vi "ZSort_Scan_Params.vi"(8 "error in (no error)":errorcluster, 11 "Sweep Metadata Cluster":T1 {"Channels: AO"."AO f (Hz)" min=0.001 max=10000.0; "Channels: AO"."AO DC (V)" format="%#_6p"; "Channels: AO"."AO amp (V)" format="%#_6p"}) -> (0 "error out":errorcluster, 1 "Sorted scan parameters":cluster{T15}[](array[cluster])=[{[{"Start"=0.14, "End"=-0.060000000000000005, "Step"=-0.060000000000000005, "Rate"=0.0, "wait (ms)"=10000, "address"="\nscaledVsg1=", "Channel"=2}]}, {[{"Start"=0.14, "End"=-0.060000000000000005, "Step"=-0.060000000000000005, "Rate"=0.0, "wait (ms)"=10000, "address"="\nscaledVsg1=", "Channel"=2}]}, {[{"Start"=0.14, "End"=-0.060000000000000005, "Step"=-0.060000000000000005, "Rate"=0.0, "wait (ms)"=10000, "address"="\nscaledVsg1=", "Channel"=2}, {"Start"=0.14, "End"=-0.060000000000000005, "Step"=-0.060000000000000005, "Rate"=0.0, "wait (ms)"=10000, "address"="\nscaledVsg1=", "Channel"=3}]}] {"?"."Rate" format="%.2f"; "?"."Step" format="%#_6p"; "?"."End" format="%#_6p"; "?"."Start" format="%#_6p"}, 2 "Sorted scan control":cluster{T11}[](array[cluster])=[{[{"Priority"=enum."Priority 0", "Scan name"=enum."DSA_Vsg2"}]}, {[{"Priority"=enum."Priority 1", "Scan name"=enum."DSA_Vamp"}]}, {[{"Priority"=enum."Priority 2", "Scan name"=enum."DSA_Vsg1"}, {"Priority"=enum."Priority 2", "Scan name"=enum."DSA_Vsg3"}]}])   [LabVIEW 2016]
uses:
  levylab_expt_transport/src/SMOs/SweepControl/Typedefs/Cluster - ScanParamters.ctl
  levylab_expt_transport/src/SMOs/SweepControl/SweepControl.lvclass
  levylab_expt_transport/src/SMOs/SweepControl/Typedefs/ScanParamters.ctl
  levylab_expt_transport/src/SMOs/SweepControl/Typedefs/Enum - Priority.ctl
  levylab_expt_transport/src/SMOs/SweepControl/Typedefs/Enum - Action.ctl
  levylab_expt_transport/src/SMOs/SweepControl/Typedefs/Cluster - ScanControl.ctl
  levylab_expt_transport/src/SMOs/SweepControl/Typedefs/ScanControl.ctl
  <userlib>/LevyLab/Lockin-Multichannel/Typedefs/AO_Amp-array.ctl
  <userlib>/LevyLab/Lockin-Multichannel/Typedefs/AO_DC-array.ctl
  <userlib>/LevyLab/Lockin-Multichannel/Typedefs/AO_phi-array.ctl
  <userlib>/LevyLab/Lockin-Multichannel/Typedefs/Function-enum.ctl
  <userlib>/LevyLab/Lockin-Multichannel/Typedefs/Function-array.ctl
  <userlib>/LevyLab/Lockin-Multichannel/Typedefs/AO_f-array.ctl
  <userlib>/LevyLab/Lockin-Multichannel/Typedefs/AO-cluster.ctl
  levylab_expt_transport/src/SMOs/SweepControl/Typedefs/Enum - PostAction.ctl
  levylab_expt_transport/src/SMOs/SweepControl/Typedefs/PostAction.ctl
  levylab_expt_transport/src/subVI/SweepMetadataV2.ctl
panel:
  # "0"
  # "1"
  # "2"
  # "3"
  # "4"
  # "5"
  # "6"
  # "7"
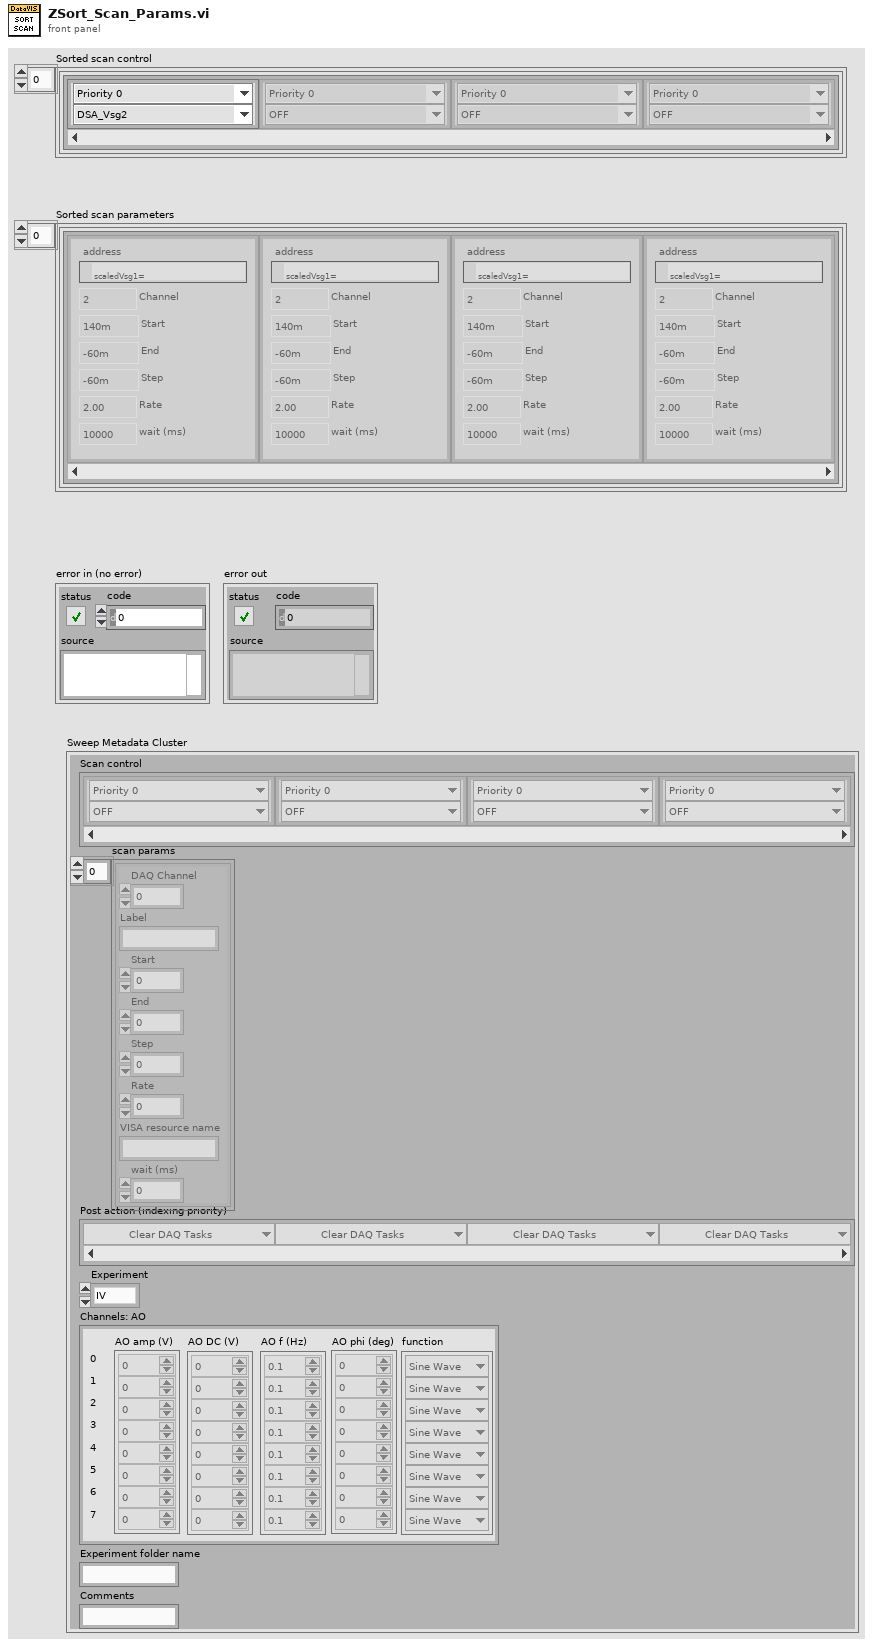
[diagram p1: front panel]
types:
  T1 = typedef "SweepMetadataV2.ctl" = cluster{"Experiment":enum16{"IV", "lockin_time", "Lockin_Vsg"}, "Experiment folder name":string, "Comments":string, "Channels: AO":T2, "Post action (indexing priority)":T9, "Scan control":T11, "scan params":cluster{"DAQ Channel":i32, "Label":string, "Start":dbl, "End":dbl, "Step":dbl, "Rate":dbl, "VISA resource name":string, "wait (ms)":u32}[]}
  T2 = typedef "AO-cluster.ctl" = cluster{"AO amp (V)":T3, "AO DC (V)":T4, "AO f (Hz)":T5, "AO phi (deg)":T6, "function":T7}
  T3 = typedef "AO_Amp-array.ctl" = dbl[]
  T4 = typedef "AO_DC-array.ctl" = dbl[]
  T5 = typedef "AO_f-array.ctl" = dbl[]
  T6 = typedef "AO_phi-array.ctl" = dbl[]
  T7 = typedef "Function-array.ctl" = T8[]
  T8 = typedef "Function-enum.ctl" = enum16{"Sine Wave", "Triangle Wave", "Square Wave", "Sawtooth Wave"}
  T9 = typedef "SweepControl.lvclass/PostAction.ctl" = T10[]
  T10 = typedef "SweepControl.lvclass/Enum - PostAction.ctl" = enum16{"Clear DAQ Tasks", "Check Temperature", "Wait", "Do Nothing"}
  T11 = typedef "SweepControl.lvclass/ScanControl.ctl" = T12[]
  T12 = typedef "SweepControl.lvclass/Cluster - ScanControl.ctl" = cluster{"Priority":T13, "Scan name":T14}
  T13 = typedef "SweepControl.lvclass/Enum - Priority.ctl" = enum16{"Priority 0", "Priority 1", "Priority 2", "Priority 3", "Priority 4", "Priority 5"}
  T14 = typedef "SweepControl.lvclass/Enum - Action.ctl" = enum16{"OFF", "DSA_Vamp", "DSA_freq", "DSA_Vsg1", "DSA_Vsg2", "DSA_Vsg3", "DAQ_Vbg", "B_Field", "Humidity", "Temp", "MW_freq1", "MW_freq2", "MW_amplitude1", "MW_amplitude2"}
  T15 = typedef "SweepControl.lvclass/ScanParamters.ctl" = T16[]
  T16 = typedef "SweepControl.lvclass/Cluster - ScanParamters.ctl" = cluster{"Start":dbl, "End":dbl, "Step":dbl, "Rate":dbl, "wait (ms)":u32, "address":refnum<visa-resource-name>, "Channel":i32}
  T17 = cluster{"DAQ Channel":i32, "Label":string, "Start":dbl, "End":dbl, "Step":dbl, "Rate":dbl, "VISA resource name":string, "wait (ms)":u32}[]
  T18 = cluster{"DAQ Channel":i32, "Label":string, "Start":dbl, "End":dbl, "Step":dbl, "Rate":dbl, "VISA resource name":string, "wait (ms)":u32}
  T19 = cluster{cluster{"DAQ Channel":i32, "Label":string, "Start":dbl, "End":dbl, "Step":dbl, "Rate":dbl, "VISA resource name":string, "wait (ms)":u32}[]}
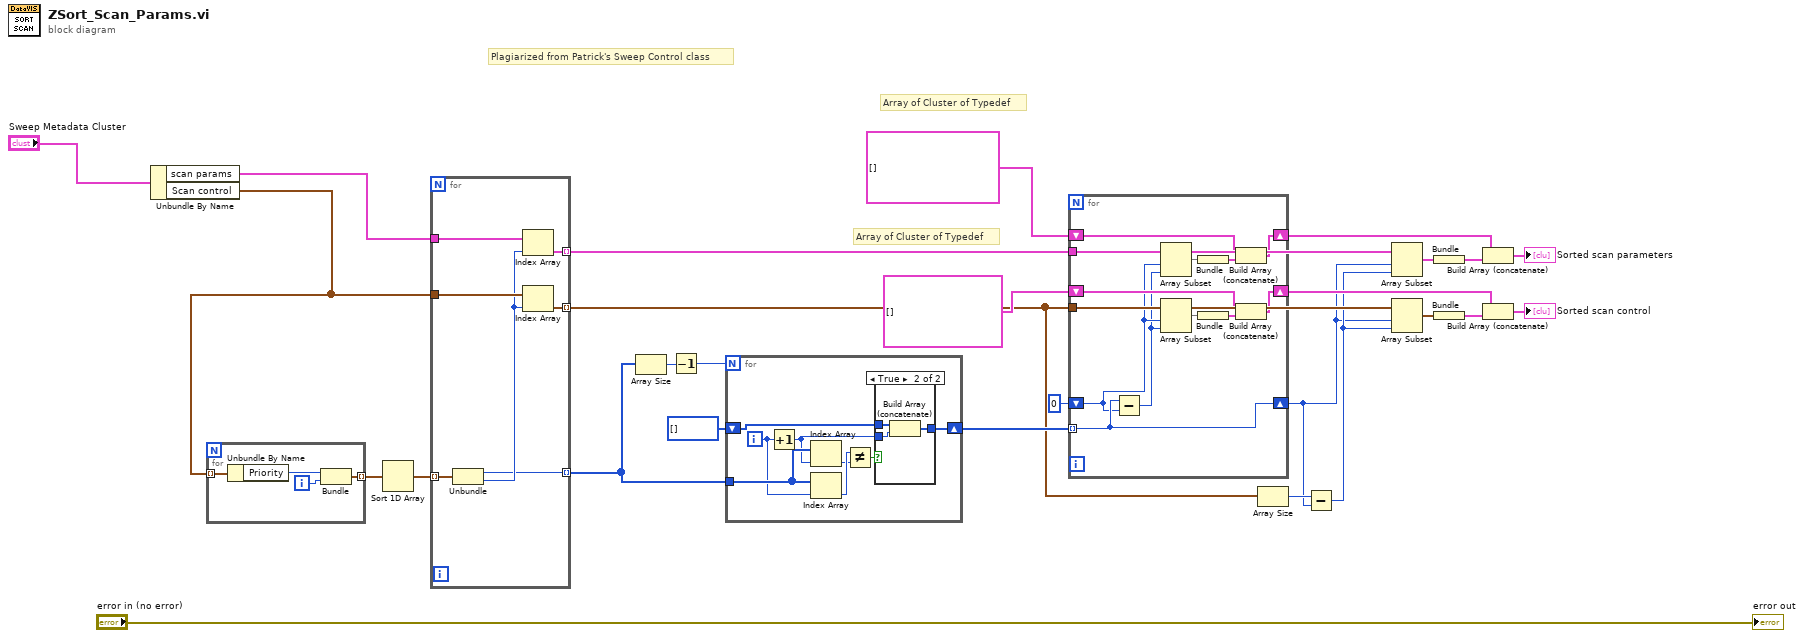
[diagram p0: block diagram]
diagram:
  # "Plagiarized from Patrick's Sweep Control class"
  # "Array of Cluster of Typedef"
  # "Array of Cluster of Typedef"
  n1 = Unbundle By Name("Sweep Metadata Cluster") -> ("scan params"=w6:T17, "Scan control"=w5:T11)
  n2 = for {
    tunnel: w5 -> [w28] mode=indexing
    tunnel: [w31] -> w27 mode=indexing
    i -> [w29]
    n3 = Unbundle By Name(w28) -> ("Priority"=w30:T13)
    n4 = Bundle("Priority"=w30, w29) -> (w31:cluster{"Priority":T13, i32})  [unwired: 1 in]
  }
  n5 = Sort 1D Array(array=w27) -> (sorted array=w26:cluster{"Priority":T13, i32}[])
  n6 = for {
    tunnel: w26 -> [w38] mode=indexing
    tunnel: w5 -> [w37]
    tunnel: [w36] -> w16 mode=indexing
    tunnel: w6 -> [w35]
    tunnel: [w34] -> w12 mode=indexing
    tunnel: [w32] -> w23 mode=indexing
    n7 = Unbundle(w38) -> ("Priority"=w32:T13, w33:i32)
    n8 = Index Array(array=w35, index=w33) -> (element=w34:T18)
    n9 = Index Array(array=w37, index=w33) -> (element=w36:T12)
  }
  n10 = Array Size(array=w23) -> (size(s)=w25:i32)
  n11 = Decrement(x=w25) -> (x-1=w24:i32)
  n12 = for {
    N: w24 -> [_]
    tunnel: w23 -> [w46]
    shift-right: [w42] -> w20
    shift-left: i32[] [] -> [w41]
    i -> [w39]
    n13 = Increment(x=w39) -> (x+1=w40:i32)
    n14 = Index Array(array=w46, index=w40) -> (element=w43:T13)
    n15 = Index Array(array=w46, index=w39) -> (element=w45:T13)
    n16 = Not Equal?(x=w45, y=w43) -> (x != y?=w44:bool)
    n17 = case shown="True" w44 {
      tunnel: [w47 w50] -> w42
      tunnel: w41 -> [w47 w49]
      tunnel: w40 -> [_ w48]
      frame False {
      }
      frame True {
        n18 = Build Array (concatenate)(w49, w48) -> (w50:i32[])
      }
    }
  }
  n19 = for {
    tunnel: w20 -> [w58] mode=indexing
    shift-right: [w63] -> w19
    shift-left: cluster{"Scan control":T11}[] [] -> [w62]
    tunnel: w16 -> [w61]
    shift-right: [w58] -> w10
    shift-left: 0 -> [w56]
    tunnel: w12 -> [w57]
    shift-right: [w53] -> w7
    shift-left: cluster{"Scan parameters":T15}[] [] -> [w52]
    n20 = Subtract(x=w58, y=w56) -> (x-y=w55:i32)
    n21 = Array Subset(array=w57, index=w56, length=w55) -> (w54:T17)
    n22 = Array Subset(array=w61, index=w56, length=w55) -> (w60:T12[])
    n23 = Bundle(w54) -> (w51:T19)  [unwired: 1 in]
    n24 = Bundle(w60) -> (w59:cluster{T12[]})  [unwired: 1 in]
    n25 = Build Array (concatenate)(w52, w51) -> (w53:cluster{"Scan parameters":T15}[])
    n26 = Build Array (concatenate)(w62, w59) -> (w63:cluster{"Scan control":T11}[])
  }
  n27 = Array Size(array=w16) -> (size(s)=w17:i32)
  n28 = Subtract(x=w17, y=w10) -> (x-y=w11:i32)
  n29 = Array Subset(array=w12, index=w10, length=w11) -> (w13:T17)
  n30 = Array Subset(array=w16, index=w10, length=w11) -> (w15:T12[])
  n31 = Bundle(w13) -> (w9:T19)  [unwired: 1 in]
  n32 = Bundle(w15) -> (w14:cluster{T12[]})  [unwired: 1 in]
  n33 = Build Array (concatenate)(w7, w9) -> (→"Sorted scan parameters":cluster{"Scan parameters":T15}[])
  n34 = Build Array (concatenate)(w19, w14) -> (→"Sorted scan control":cluster{"Scan control":T11}[])
  "error out" <- "error in (no error)"
